vi "ResetCollectionConditions.vi"(7 "dg_op":string, 8 "error in (no error)":errorcluster, 9 "ConditionType":T1, 10 "snapshot map":T2, 11 "operating states in":variant) -> (0 "error out":errorcluster, 3 "operating states out":variant)   [LabVIEW 2017, in "Trigger.lvlib"]
uses:
  <vilib>/addons/InsightCM/Devices/Shared/Common/Trigger/Trigger.lvlib
  <vilib>/addons/PointValueMap/controls/PointMap.ctl
  <vilib>/addons/InsightCM/Devices/Shared/Common/Trigger/controls/ConditionType.ctl
  <vilib>/addons/InsightCM/Devices/Shared/Common/Trigger/controls/TriggerOperatingState.ctl
  <vilib>/addons/InsightCM/MessageBus/Base/controls/KeyValuePair.ctl
  <vilib>/addons/InsightCM/Devices/Shared/Common/Trigger/controls/TriggerCondition.ctl
  <vilib>/addons/InsightCM/MessageBus/Base/controls/Condition.ctl
  <vilib>/addons/PointValueMap/PointValueMap.lvlib
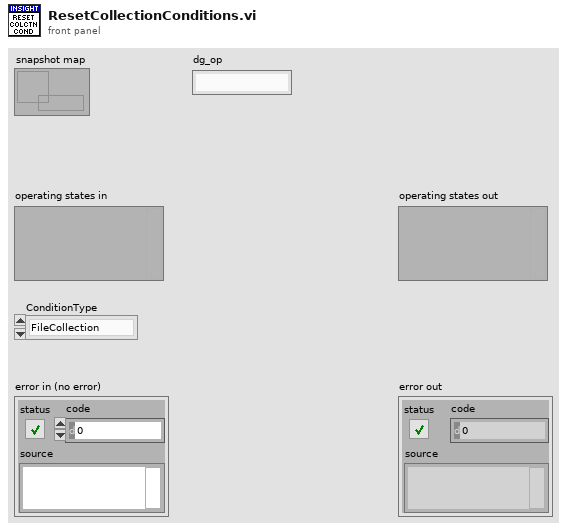
[diagram p1: front panel]
types:
  T1 = typedef "Trigger.lvlib/ConditionType.ctl" = enum16{"FileCollection", "TrendCollection"}
  T2 = typedef "PointValueMap.lvlib/PointMap.ctl" = refnum<data-value>
  T3 = typedef "Trigger.lvlib/TriggerOperatingState.ctl" = cluster{"Id":string, "Name":string, "Properties":T4[], "TrendExpression":string, "TrendConditions":T5[], "FileExpression":string, "FileConditions":T5[]}
  T4 = typedef "KeyValuePair.ctl" = cluster{"Key":string, "Value":string}
  T5 = typedef "Trigger.lvlib/TriggerCondition.ctl" = cluster{"Condition":T6, "LatchValue":string, "LatchTime":timestamp}
  T6 = typedef "Condition.ctl" = cluster{"Source":string, "Type":string, "Operator":string, "CompareTo":string, "DwellSeconds":dbl}
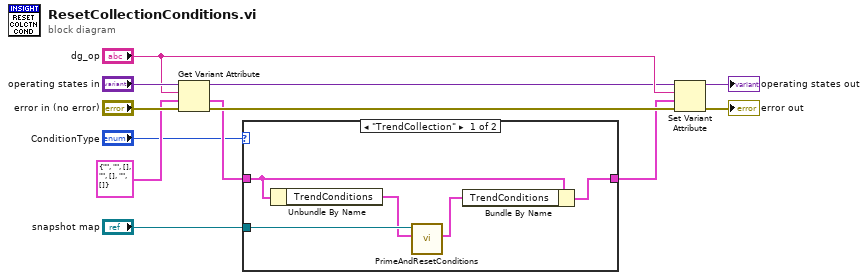
[diagram p0: block diagram]
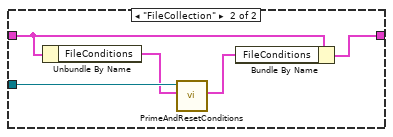
[diagram p2: hidden frame]
diagram:
  n1 = Get Variant Attribute(Variant="operating states in", name="dg_op", default value (empty Variant)=T3 {"Id"="", "Name"="", "Properties"=[], "TrendExpression"="", "TrendConditions"=[], "FileExpression"="", "FileConditions"=[]} ("OperatingState"), error in="error in (no error)") -> (duplicate Variant=w7:variant, value=w3:T3, error out=w10:errorcluster)  [unwired: 1 out]
  n2 = case shown="\"TrendCollection\"" "ConditionType" {
    tunnel: "snapshot map" -> [w17 w22]
    tunnel: w3 -> [w14 w19]
    tunnel: [w13 w18] -> w2
    frame "TrendCollection" {
      n3 = Unbundle By Name(w14) -> ("TrendConditions"=w16:T5[])
      n4 = call <vilib>:"PrimeAndResetConditions.vi"("conditions in"=w16, "SnapshotMap"=w17) -> ("conditions out"=w15:T5[])  [unwired: 8 in, 1 out]
      n5 = Bundle By Name(cluster=w14, "TrendConditions"=w15) -> (w13:T3)
    }
    frame "FileCollection" {
      n6 = Unbundle By Name(w19) -> ("FileConditions"=w21:T5[])
      n7 = call <vilib>:"PrimeAndResetConditions.vi"("conditions in"=w21, "SnapshotMap"=w22) -> ("conditions out"=w20:T5[])  [unwired: 8 in, 1 out]
      n8 = Bundle By Name(cluster=w19, "FileConditions"=w20) -> (w18:T3)
    }
  }
  n9 = Set Variant Attribute(Variant=w7, name="dg_op", value=w2, error in=w10) -> (Variant out=→"operating states out":variant, error out=→"error out":errorcluster)  [unwired: 1 out]
